vi "Single SMU SENSE Pins.vi"(8 "error in":errorcluster, 11 "TSM context":T1) -> (0 "error out":errorcluster)   [LabVIEW 2019]
uses:
  <vilib>/NI_TestStand_SemiconductorModule/NI_TestStand_Semiconductor_Module.lvlibp/PinMap/General/SemiconductorModuleContext.ctl
  <vilib>/NI_TestStand_SemiconductorModule/NI_TestStand_Semiconductor_Module.lvlibp/1abvi3w/instr.lib/niSwitch/niswitch.llb/niSwitch Relay Action.ctl
  <vilib>/NI_TestStand_SemiconductorModule/NI_TestStand_Semiconductor_Module.lvlibp
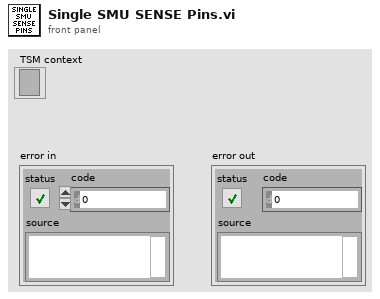
[diagram p1: front panel]
types:
  T1 = typedef "NI_TestStand_Semiconductor_Module.lvlibp/SemiconductorModuleContext.ctl" = refnum<k7>
  T2 = typedef "NI_TestStand_Semiconductor_Module.lvlibp/niSwitch Relay Action.ctl" = i32
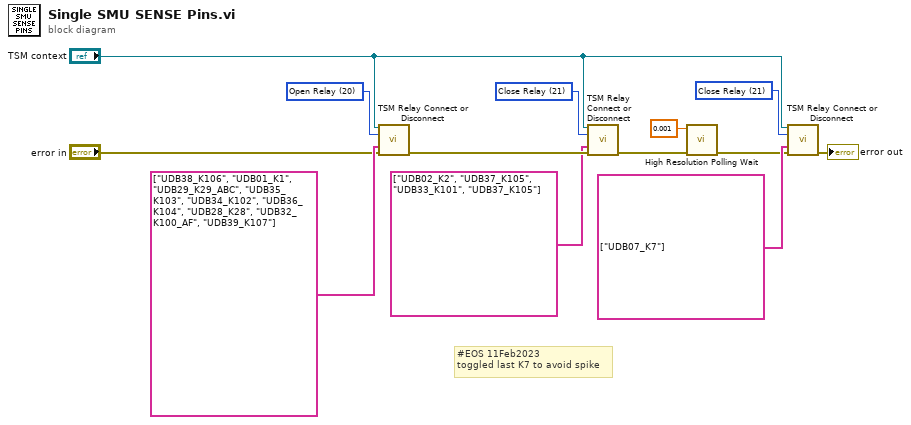
[diagram p0: block diagram]
diagram:
  w7 = T2 21 items=["Open Relay"=20, "Close Relay"=21] ("Relay Action")
  w10 = T2 21 items=["Open Relay"=20, "Close Relay"=21] ("Relay Action")
  w13 = T2 20 items=["Open Relay"=20, "Close Relay"=21] ("Relay Action")
  # "#EOS 11Feb2023\ntoggled last K7 to avoid spike"
  n1 = call "TSM Relay Connect or Disconnect.vi"("TSM context"="TSM context", "Relay Action"=w13, "Relays"=tag[] ["UDB38_K106", "UDB01_K1", "UDB29_K29_ABC", "UDB35_K103", "UDB34_K102", "UDB36_K104", "UDB28_K28", "UDB32_K100_AF", "UDB39_K107"], "error in"="error in") -> ("error out"=w9:errorcluster)  [unwired: 10 in, 1 out]
  n2 = call "TSM Relay Connect or Disconnect.vi"("TSM context"="TSM context", "Relay Action"=w10, "Relays"=tag[] ["UDB02_K2", "UDB37_K105", "UDB33_K101", "UDB37_K105"], "error in"=w9) -> ("error out"=w6:errorcluster)  [unwired: 10 in, 1 out]
  n3 = call <vilib>:"High Resolution Polling Wait.vi"("error in (no error)"=w6, "seconds to wait"=0.001) -> ("error out"=w2:errorcluster)  [unwired: 9 in]
  n4 = call "TSM Relay Connect or Disconnect.vi"("TSM context"="TSM context", "Relay Action"=w7, "Relays"=tag[] ["UDB07_K7"], "error in"=w2) -> ("error out"=→"error out":errorcluster)  [unwired: 10 in, 1 out]
